vi "Parse Headers.vi"(8 "error in (no error)":errorcluster, 10 "String in":string, 11 "Request in":refnum<class "Request.lvclass">) -> (0 "error out":errorcluster, 3 "Request out":refnum<class "Request.lvclass">)   [LabVIEW 2020, in "HTTP Utils.lvlib" / "Request.lvclass"]
uses:
  Request.lvclass
  Request.lvclass/Request.ctl
  <vilib>/IlluminatedG/lv-stream/Stream.lvlib
  Cookie/Cookie.lvclass
  Cookie Map.ctl
  HTTP Utils.lvlib
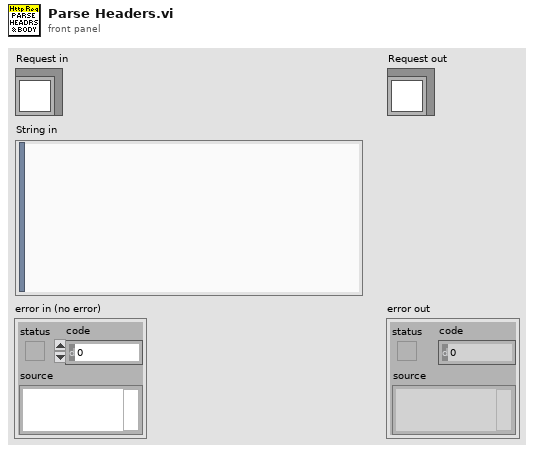
[diagram p1: front panel]
types:
  T1 = typedef "HTTP Utils.lvlib/Cookie Map.ctl" = map{string, refnum<class "Cookie.lvclass">}
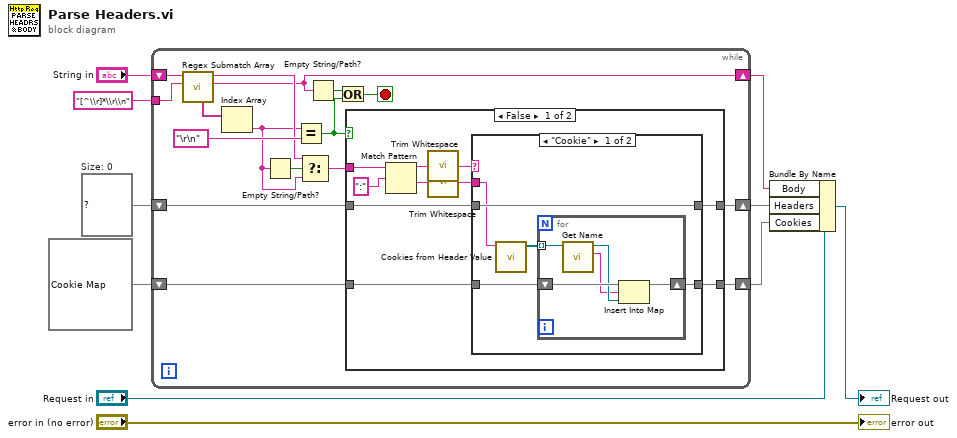
[diagram p0: block diagram]
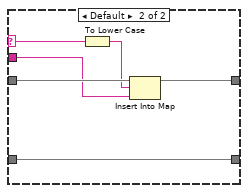
[diagram p2: hidden frame]
diagram:
  w8 = map{string, string} {}  # Size: 0
  n1 = while {
    shift-right: [w15] -> w1
    shift-left: "String in" -> [w18]
    shift-right: [w25] -> w6
    shift-left: w8 -> [w26]
    tunnel: "[^\\r]*\\r\\n" ("regular expression") -> [w17]
    shift-right: [w11] -> w2
    shift-left: T1 {} ("Cookies") -> [w12]
    stop <- w21 stop-if-true
    n2 = call <vilib>:"Regex Submatch Array.vi"("regular expression"=w17, "string"=w18) -> ("after match"=w15:string, "before match"=w16:string, "matches"=w14:string[])  [unwired: 5 in, 2 out]
    n3 = Index Array(array=w14) -> (element=w13:string)  [unwired: 1 in]
    n4 = Empty String/Path?(string/path=w13) -> (empty?=w20:bool)
    n5 = Equal?(x=w13, y="\r\n" ("regular expression")) -> (x = y?=w22:bool)
    n6 = Select(t=w16, s=w20, f=w13) -> (s? t:f=w19:string)
    n7 = Empty String/Path?(string/path=w15) -> (empty?=w23:bool)
    n8 = Or(x=w23, y=w22) -> (x .or. y?=w21:bool)
    n9 = case shown="False" w22 {
      tunnel: w19 -> [w35 _]
      tunnel: w26 -> [w36 w54]
      tunnel: [w33 w54] -> w25
      tunnel: w12 -> [w28 w53]
      tunnel: [w27 w53] -> w11
      frame False {
        n10 = Match Pattern(string=w35, regular expression=":") -> (before substring=w32:string, after substring=w30:string)  [unwired: 1 in, 2 out]
        n11 = call <vilib>:"Trim Whitespace.vi"("string"=w32) -> ("trimmed string"=w31:string)  [unwired: 1 in]
        n12 = call <vilib>:"Trim Whitespace.vi"("string"=w30) -> ("trimmed string"=w29:string)  [unwired: 1 in]
        n13 = case shown="\"Cookie\"" w31 {
          selector: w31 -> [_ w49]
          tunnel: w36 -> [w41 w52]
          tunnel: [w41 w50] -> w33
          tunnel: w29 -> [w40 w48]
          tunnel: w28 -> [w38 w47]
          tunnel: [w37 w47] -> w27
          frame "Cookie" {
            n14 = call "Cookies from Header Value.vi"("Cookie Header Value"=w40) -> ("Cookies"=w39:refnum<class "Cookie.lvclass">[])  [unwired: 9 in, 1 out]
            n15 = for {
              tunnel: w39 -> [w46] mode=indexing
              shift-right: [w42] -> w37
              shift-left: w38 -> [w45]
              n16 = call "Get Name.vi"("Cookie in"=w46) -> ("Name"=w43:string, "Cookie out"=w44:refnum<class "Cookie.lvclass">)  [unwired: 8 in, 1 out]
              n17 = Insert Into Map(map in=w45, key=w43, value=w44) -> (map out=w42:T1)  [unwired: 2 out]
            }
          }
          frame Default {
            n18 = To Lower Case(string=w49) -> (all lower case string=w51:string)
            n19 = Insert Into Map(map in=w52, key=w51, value=w48) -> (map out=w50:map{string, string})  [unwired: 2 out]
          }
        }
      }
      frame True {
      }
    }
  }
  n20 = Bundle By Name(cluster="Request in", "Body"=w1, "Headers"=w6, "Cookies"=w2) -> (→"Request out":refnum<class "Request.lvclass">)
  "error out" <- "error in (no error)"
